vi "leebinario_calibracion.vi"() -> ()   [LabVIEW 2015]
uses:
  <vilib>/measure/maspectr.llb/FFT Spectrum (Mag-Phase) for 1 Chan.vi
  <vilib>/measure/NI_MAPro.lvlib
panel:
  out "Frecuencia de excitación\nVibrómetro  (Hz)":dbl
  out "f PRINCIPAL":dbl
  out "magnitude":cluster{"f0":dbl, "df":dbl, "magnitude":dbl[]} {"magnitude" format="%.2p"; "f0" format="%0.2p"; "df" format="%0.2p"}
  in  "CANAL FFT":i32
  in  "Nº canales":i32=10
  out "size(s) 2":i32
  out "Waveform Graph":waveform(sgl)[](graph)
  in  "Folder Path":path
  out "error out":errorcluster
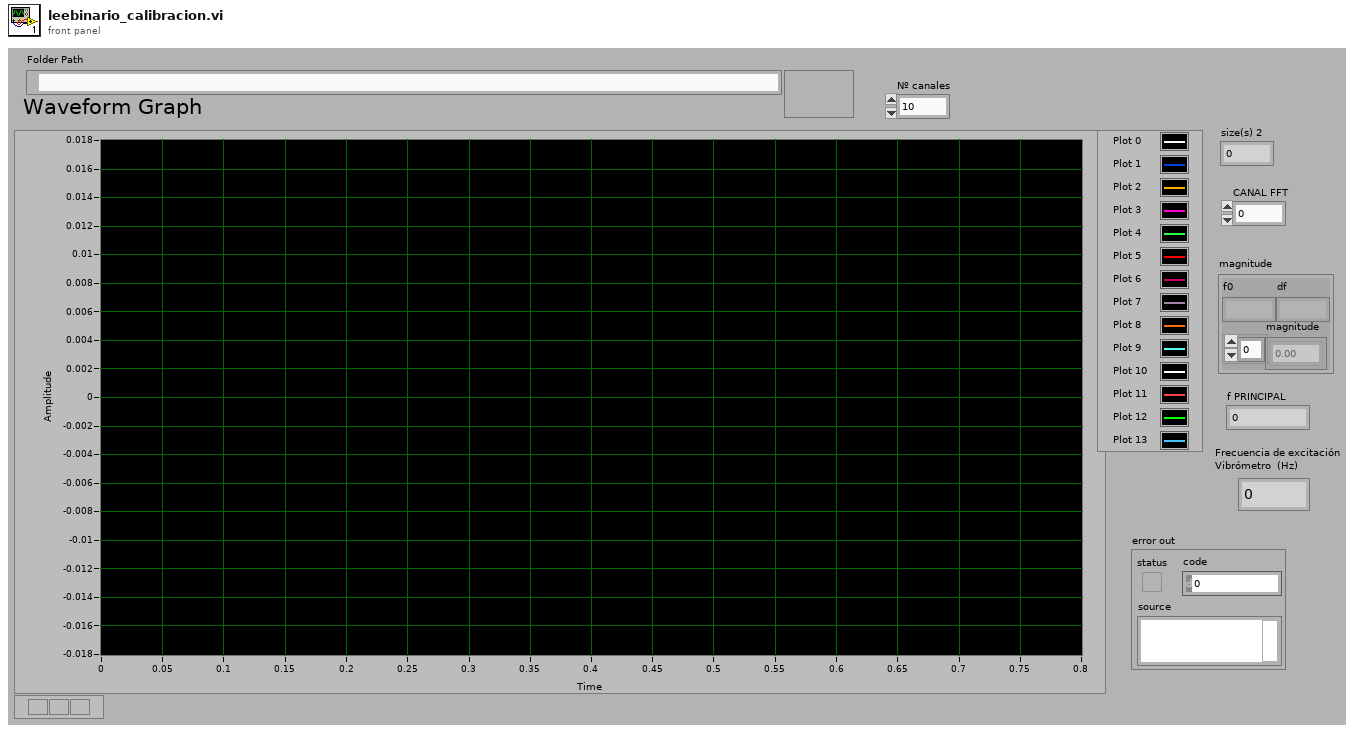
[diagram p1: front panel]
types:
  T1 = enum16{"big-endian, network order", "native, host order", "little-endian"}
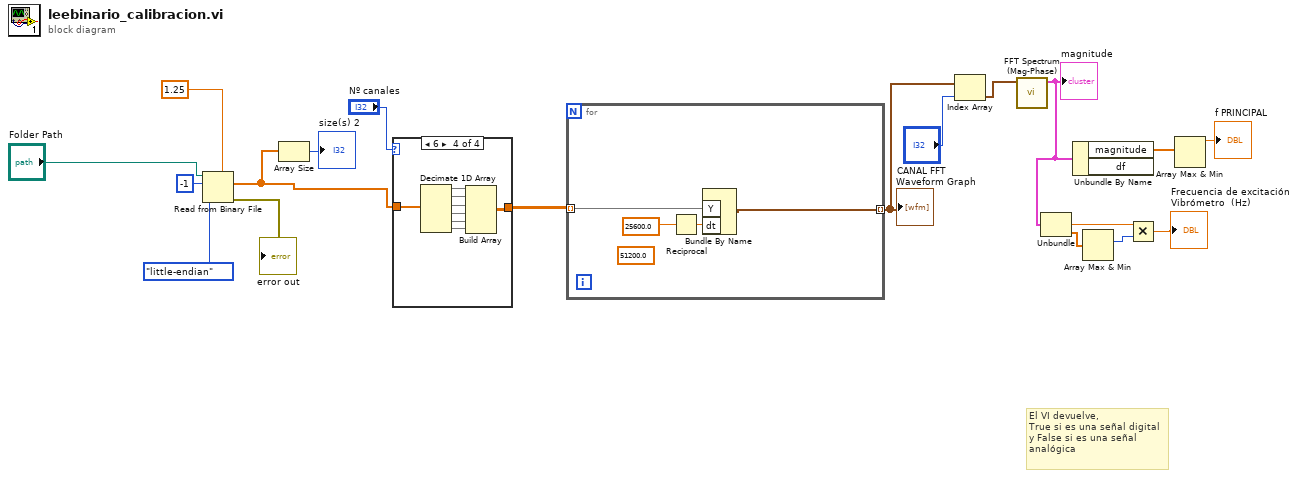
[diagram p0: block diagram]
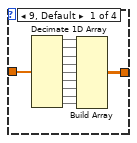
[diagram p2: hidden frame]
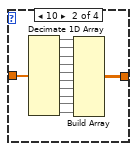
[diagram p3: hidden frame]
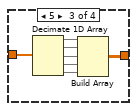
[diagram p4: hidden frame]
diagram:
  # "El VI devuelve,\nTrue si es una señal digital\ny False si es una señal\nanalógica"
  n1 = Read from Binary File(5:sgl 1.25, 9:T1."little-endian" ("byte order (0:big-endian, network order)"), 10:-1 ("count (1)"), 11:"Folder Path") -> (0:→"error out":errorcluster, 2:w12:sgl[])  [unwired: 1 in, 3 out]
  n2 = Array Size(array=w12) -> (size(s)=→"size(s) 2":i32)
  n3 = case shown="6" "Nº canales" {
    tunnel: [w20 w33 w43 w51] -> w11
    tunnel: w12 -> [w21 w31 w44 w52]
    frame 9, Default {
      n4 = Decimate 1D Array(w21) -> (w22:sgl[], w30:sgl[], w29:sgl[], w25:sgl[], w24:sgl[], w26:sgl[], w27:sgl[], w28:sgl[], w23:sgl[])
      n5 = Build Array(w22, w30, w29, w25, w24, w26, w27, w28, w23) -> (w20:sgl[][])
    }
    frame 10 {
      n6 = Decimate 1D Array(w31) -> (w32:sgl[], w42:sgl[], w41:sgl[], w37:sgl[], w36:sgl[], w38:sgl[], w39:sgl[], w40:sgl[], w35:sgl[], w34:sgl[])
      n7 = Build Array(w32, w42, w41, w37, w36, w38, w39, w40, w35, w34) -> (w33:sgl[][])
    }
    frame 5 {
      n8 = Decimate 1D Array(w44) -> (w45:sgl[], w49:sgl[], w48:sgl[], w47:sgl[], w46:sgl[])
      n9 = Build Array(w45, w49, w48, w47, w46) -> (w43:sgl[][])
    }
    frame 6 {
      n10 = Decimate 1D Array(w52) -> (w57:sgl[], w53:sgl[], w54:sgl[], w55:sgl[], w56:sgl[], w50:sgl[])
      n11 = Build Array(w57, w53, w54, w55, w56, w50) -> (w51:sgl[][])
    }
  }
  n12 = for {
    tunnel: [w61] -> w10 mode=indexing
    tunnel: w11 -> [w59] mode=indexing
    (unwired) 51200.0 ("dt")
    n13 = Reciprocal(x=25600.0 ("dt")) -> (1/x=w60:dbl)
    n14 = Bundle By Name("Y"=w59, "dt"=w60) -> (w61:waveform(sgl))  [unwired: 1 in]
  }
  "Waveform Graph" <- w10
  n15 = Index Array(array=w10, index="CANAL FFT") -> (element=w8:waveform(sgl))
  n16 = call-poly <vilib>:"FFT Spectrum (Mag-Phase).vi"("time signal"=w8) -> ("magnitude"=w1:cluster{"f0":dbl, "df":dbl, "magnitude":dbl[]})  [unwired: 6 in, 4 out]
  "magnitude" <- w1
  n17 = Unbundle(w1) -> ("df"=w3:dbl, "magnitude"=w4:dbl[])  [unwired: 1 out]
  n18 = Unbundle By Name(w1) -> ("magnitude"=w7:dbl[])  [unwired: 1 out]
  n19 = Array Max & Min(array=w4) -> (max index (indices)=w5:i32)  [unwired: 3 out]
  n20 = Multiply(x=w3, y=w5) -> (x*y=→"Frecuencia de excitación\nVibrómetro  (Hz)":dbl)
  n21 = Array Max & Min(array=w7) -> (max value=→"f PRINCIPAL":dbl)  [unwired: 3 out]
